vi "Lint Owned Items.vi"(8 "Error In":errorcluster, 11 "Owned Items In":refnum<vi>[](array[refnum])) -> (0 "Error Out":errorcluster, 2 "Results":T1[](array[typedef]), 3 "Owned Items Out":refnum<vi>[](array[refnum]))   [LabVIEW 2018, in "Scripts.lvlib"]
uses:
  Scripts.lvlib
  Project Item Lint Result.ctl
  VI Control Lint Result.ctl
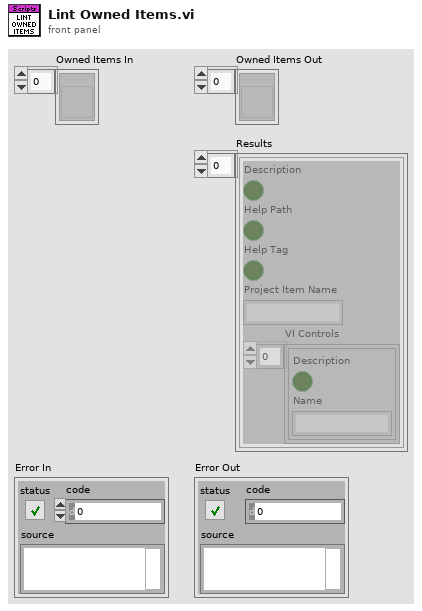
[diagram p1: front panel]
types:
  T1 = typedef "Scripts.lvlib/Project Item Lint Result.ctl" = cluster{"Description":bool, "Help Path":bool, "Help Tag":bool, "Project Item Name":string, "VI Controls":T2[]}
  T2 = typedef "Scripts.lvlib/VI Control Lint Result.ctl" = cluster{"Description":bool, "Name":string}
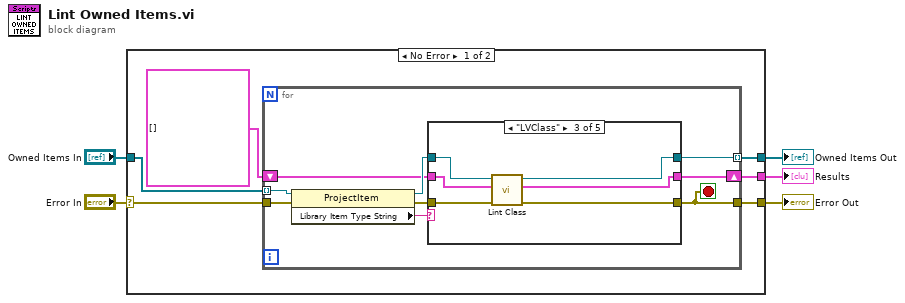
[diagram p0: block diagram]
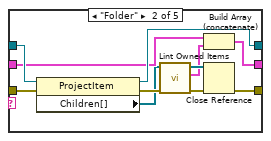
[diagram p3: hidden frame]
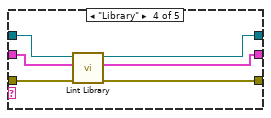
[diagram p4: hidden frame]
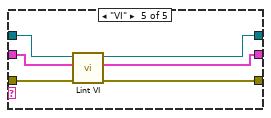
[diagram p5: hidden frame]
diagram:
  n1 = case shown="No Error" "Error In" {
    selector: "Error In" -> [w8 w53]
    tunnel: "Owned Items In" -> [w11 w54]
    tunnel: [w10 w54] -> w4
    tunnel: [w9 w53] -> w3
    tunnel: [w6 _] -> w1
    frame No Error {
      n2 = for {
        tunnel: w11 -> [w20] mode=indexing
        tunnel: w8 -> [w19]
        tunnel: [w16] -> w10 mode=indexing
        tunnel: [w14] -> w9
        shift-right: [w12] -> w6
        shift-left: T1[] [] ("Results") -> [w13]
        stop <- w14 stop-if-true
        n3 = property class="ProjectItem"(reference=w20, error in=w19) -> (reference out=w17:refnum<vi>, error out=w15:errorcluster, "Library Item Type String"=w18:string)
        n4 = case shown="\"LVClass\"" w18 {
          tunnel: w15 -> [w22 w33 w40 w46 w51]
          tunnel: w17 -> [w23 w34 w38 w44 w52]
          tunnel: [w23 w32 w37 w43 w47] -> w16
          tunnel: [w22 w31 w39 w45 w50] -> w14
          tunnel: w13 -> [w21 w30 w36 w42 w49]
          tunnel: [w21 w29 w35 w41 w48] -> w12
          frame "", Default {
          }
          frame "Folder" {
            n5 = property class="ProjectItem"(reference=w34, error in=w33) -> (reference out=w32:refnum<vi>, error out=w26:errorcluster, "Children[]"=w25:refnum<vi>[])
            n6 = call "Lint Owned Items.vi"("Error In"=w26, "Owned Items In"=w25) -> ("Error Out"=w28:errorcluster, "Results"=w24:T1[], "Owned Items Out"=w27:refnum<vi>[])  [unwired: 7 in]
            n7 = Build Array (concatenate)(w30, w24) -> (w29:T1[])
            n8 = Close Reference(reference=w27, error in (no error)=w28) -> (error out=w31:errorcluster)
          }
          frame "LVClass" {
            n9 = call "Lint Class.vi"("Error In"=w40, "Results In"=w36, "Project Item In"=w38) -> ("Error Out"=w39:errorcluster, "Results Out"=w35:T1[], "Project Item Out"=w37:refnum<vi>)  [unwired: 6 in]
          }
          frame "Library" {
            n10 = call "Lint Library.vi"("Error In"=w46, "Results In"=w42, "Project Item In"=w44) -> ("Error Out"=w45:errorcluster, "Results Out"=w41:T1[], "Project Item Out"=w43:refnum<vi>)  [unwired: 6 in]
          }
          frame "VI" {
            n11 = call "Lint VI.vi"("Error In"=w51, "Results In"=w49, "Project Item In"=w52) -> ("Error Out"=w50:errorcluster, "Results Out"=w48:T1[], "Project Item Out"=w47:refnum<vi>)  [unwired: 6 in]
          }
        }
      }
    }
    frame Error {
    }
  }
  "Owned Items Out" <- w4
  "Error Out" <- w3
  "Results" <- w1
